vi "DI Scope.vi"(8 "error in (no error)":errorcluster, 11 "Node Ptr":T3 format="%.0x") -> (0 "error out":errorcluster)   [LabVIEW 2016, in "DCM System Explorer.lvlib"]
uses:
  DCM System Explorer.lvlib
  <vilib>/NI Veristand/Custom Device API/Custom Device Item Ref.ctl
  <vilib>/Powertrain Controls/Device Drivers/DCM/Rev0/FPGA/DI - ADC Signals.ctl
  <vilib>/Powertrain Controls/Device Drivers/DCM/DI/FPGA/Capture Event.ctl
  Shared/DCM Constants and GUIDs.vi
  <vilib>/NI Veristand/Custom Device Tools/Custom Device Utility Library/NI VeriStand - Search for Item by Name.vi
  <vilib>/NI VeriStand/Custom Device API/Custom Device API.lvlib
  DCM Shared.lvlib
  <vilib>/NI Veristand/Custom Device Tools/Custom Device Utility Library/Custom Device Utility Library.lvlib
  <vilib>/Powertrain Controls/Device Drivers/DCM/Rev0/FPGA/DCM - FPGA.lvlib
  <vilib>/Powertrain Controls/Device Drivers/DCM/DI/FPGA/DCM - FPGA - DI.lvlib
panel:
  in  "Capture Length":dbl caption="[s]"
  in  "Capture Enable":bool
  in  "Capture Event":T1
  in  "DI-ADC4-Select":T2 caption="Channel Select 4"
  in  "DI-ADC3-Select":T2 caption="Channel Select 3"
  in  "DI-ADC2-Select":T2 caption="Channel Select 2"
  in  "DI-ADC1-Select":T2 caption="Channel Select 1"
  in  "Header":cluster{"Section Name":string}={"Section Name"="DI Scope Initial Settings"}
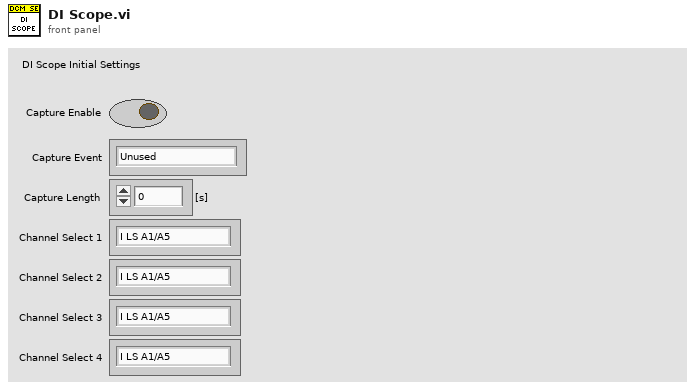
[diagram p1: front panel]
types:
  T1 = typedef "DCM - FPGA - DI.lvlib/Capture Event.ctl" = enum8{"Unused", "Injector A1", "Injector A2", "Injector A3", "Injector A4", "Injector A5", "Injector A6", "Injector A7", "Injector A8/PumpA", "Injector B1", "Injector B2", "Injector B3", "Injector B4", "Injector B5", "Injector B6", "Injector B7", "Injector B8/PumpB", "User OS", "Diff IO 1", "Diff IO 2", "Diff IO 3", "Diff IO 4", "Diff IO 5", "Diff IO 6", "Diff IO 7", "Diff IO 8", "Aux 1", "Aux 2", "Aux 3", "Aux 4", "Aux 5", "Aux 6", "Aux 7", "Aux 8", "Aux 9", "Aux 10", "Aux 11", "Aux 12", "Aux 13", "Aux 14", "Aux 15", "Aux 16"}
  T2 = typedef "DCM - FPGA.lvlib/DI - ADC Signals.ctl" = enum8{"I LS A1/A5", "I LS A2/A6", "I LS A3/A7", "I LS A4", "I LS A8/PumpA", "V PZ A1", "V PZ A2", "V PZ A3", "V PZ A4", "V S A1", "V S A2", "V S A3", "V S A4", "V S A5", "V S A6", "V S A7", "V S A8", "V Pump A", "V Secondary A1A2", "V Secondary A3A4", "V Ext HV A", "------------------------ ", "I LS B1/B5", "I LS B2/B6", "I LS B3/B7", "I LS B4", "I LS B8/PumpB", "V PZ B1", "V PZ B2", "V PZ B3", "V PZ B4", "V S B1", "V S B2", "V S B3", "V S B4", "V S B5", "V S B6", "V S B7", "V S B8", "V Pump B", "V Secondary B1B2", "V Secondary B3B4", "V Ext HV B", "-------------------------  ", "AI 1", "AI 2", "AI 3", "AI 4", "AI 5", "AI 6", "AI 7", "AI 8", "AI 9", "AI 10", "AI 11", "AI 12", "-------------------------   ", "V DRVP"}
  T3 = typedef "Custom Device API.lvlib/Custom Device Item Ref.ctl" = u64
  T4 = typedef "DCM Shared.lvlib/Channel.ctl" = cluster{"Name":string, "Units":string, "Default":dbl, "Description":string}
  T5 = typedef "Custom Device API.lvlib/Custom Device Channel.ctl" = cluster{"Type":T6, "Units":string, "Default Value":dbl, "Faultable":bool, "Scalable":bool}
  T6 = typedef "Custom Device API.lvlib/Custom Device Channel Type.ctl" = enum16{"Input", "Output"}
  T7 = typedef "Custom Device API.lvlib/Custom Device Commands.ctl" = enum16{"Default", "Item renamed", "Shutdown", "Dynamic button pressed"}
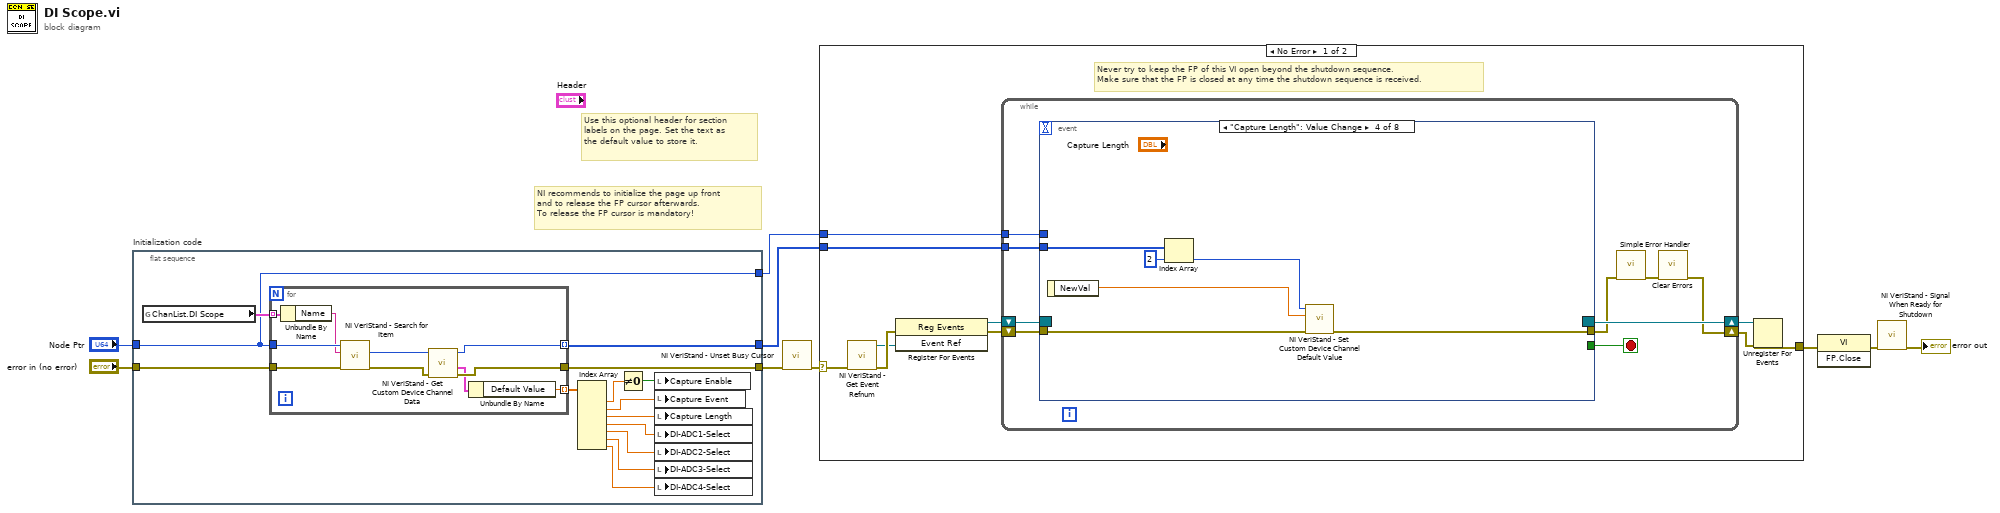
[diagram p0: block diagram]
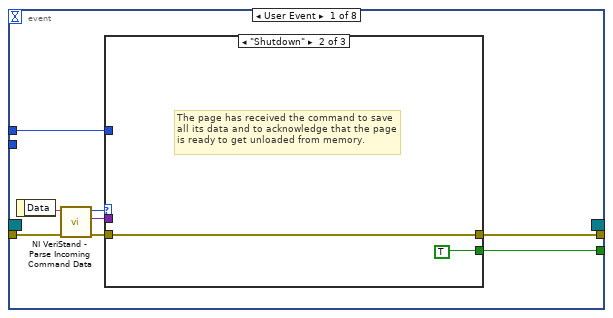
[diagram p2: hidden frame]
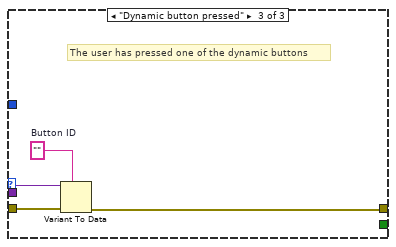
[diagram p4: hidden frame]
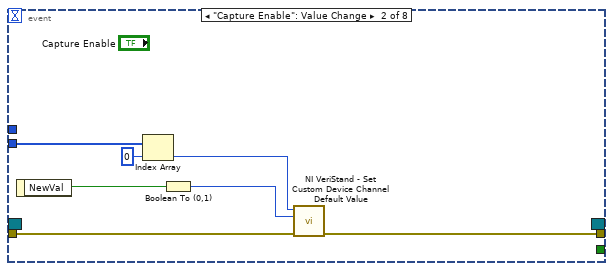
[diagram p5: hidden frame]
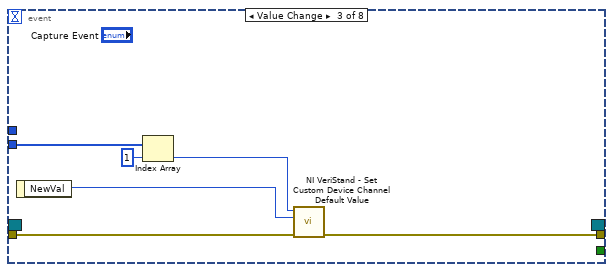
[diagram p6: hidden frame]
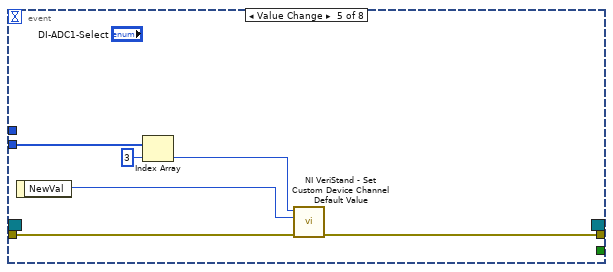
[diagram p7: hidden frame]
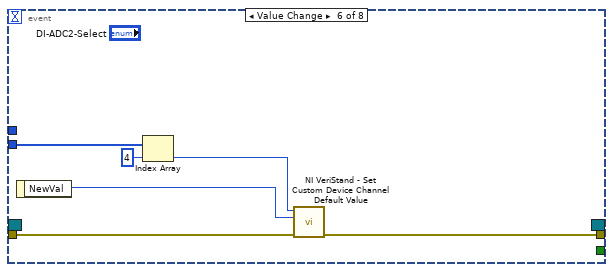
[diagram p8: hidden frame]
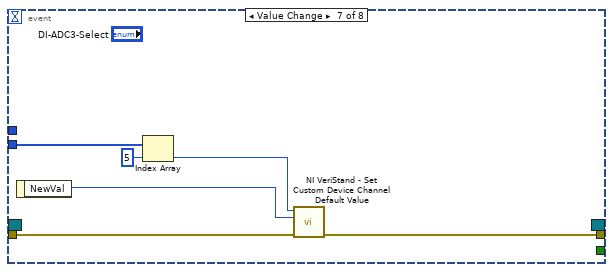
[diagram p9: hidden frame]
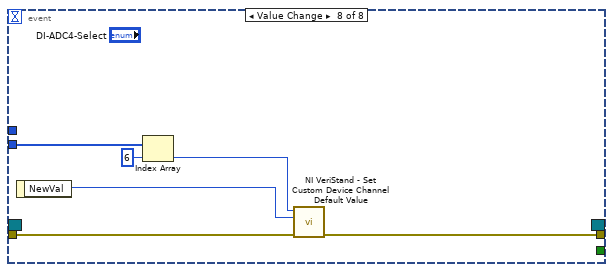
[diagram p10: hidden frame]
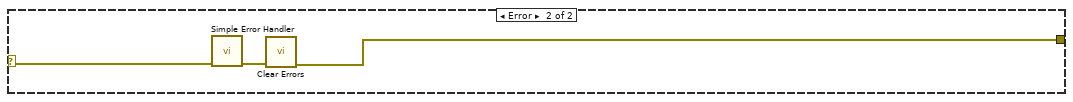
[diagram p11: hidden frame]
diagram:
  # "Use this optional header for section labels on the page. Set the text as the default value to store it."
  # "NI recommends to initialize the page up front\nand to release the FP cursor afterwards.\nTo release the FP cursor is mandatory!"
  n1 = flat-sequence "Initialization code" {
    tunnel: "error in (no error)" -> [w18]
    tunnel: "Node Ptr" -> [w16]
    tunnel: [w23] -> w5
    tunnel: [w17] -> w2
    tunnel: [w16] -> w1
    frame #0 {
      n2 = global read "DCM Constants and GUIDs.vi" "ChanList.DI Scope"() -> (w21:T4[])
      n3 = for {
        tunnel: w16 -> [w33]
        tunnel: w18 -> [w32]
        tunnel: [w24] -> w17 mode=indexing
        tunnel: [w30] -> w23
        tunnel: [w28] -> w22 mode=indexing
        tunnel: w21 -> [w27] mode=indexing
        n4 = Unbundle By Name(w27) -> ("Name"=w26:string)
        n5 = call-poly <vilib>:"NI VeriStand - Search for Item.vi"("error in"=w32, "Item Name"=w26, "Section Ref in"=w33) -> ("error out"=w31:errorcluster, "Item Ref"=w25:T3)  [unwired: 5 in, 2 out]
        n6 = call <vilib>:"NI VeriStand - Get Custom Device Channel Data.vi"("error in (no error)"=w31, "Channel Ref in"=w25) -> ("error out"=w30:errorcluster, "Channel"=w29:T5, "Channel Ref out"=w24:T3)  [unwired: 4 in, 3 out]
        n7 = Unbundle By Name(w29) -> ("Default Value"=w28:dbl)
      }
      n8 = Index Array(array=w22) -> (element #1=w12:dbl, element #2=w11:dbl, element #3=w10:dbl, element #4=w13:dbl, element #5=w15:dbl, element #6=w20:dbl, element #7=w19:dbl)  [unwired: 7 in]
      n9 = Not Equal To 0?(x=w12) -> (x != 0?=w14:bool)
      n10 = local write "Capture Enable"(w14) -> ()
      n11 = local write "Capture Event"(w11) -> ()
      n12 = local write "Capture Length"(w10) -> ()
      n13 = local write "DI-ADC1-Select"(w13) -> ()
      n14 = local write "DI-ADC2-Select"(w15) -> ()
      n15 = local write "DI-ADC3-Select"(w20) -> ()
      n16 = local write "DI-ADC4-Select"(w19) -> ()
    }
  }
  n17 = call <vilib>:"NI VeriStand - Unset Busy Cursor.vi"("error in (no error)"=w5) -> ("error out"=w4:errorcluster)  [unwired: 10 out]
  n18 = case shown="No Error" w4 {
    selector: w4 -> [w35 w113]
    tunnel: [w40 w111] -> w9
    tunnel: w2 -> [w36 _]
    tunnel: w1 -> [w34 _]
    frame No Error {
      # "Never try to keep the FP of this VI open beyond the shutdown sequence.\nMake sure that the FP is closed at any time the shutdown sequence is received."
      n19 = call <vilib>:"NI VeriStand - Get Event Refnum.vi"("error in (no error)"=w35) -> ("error out"=w43:errorcluster, "Event Ref"=w39:refnum<user-event>)  [unwired: 9 out]
      n20 = register-events(error in=w43, w39) -> (reference out=w37:refnum<event-registration>, error out=w38:errorcluster)  [unwired: 1 in]
      n21 = while {
        tunnel: w36 -> [w48]
        shift-right: [w45] -> w41
        shift-left: w38 -> [w51]
        shift-right: [w52] -> w42
        shift-left: w37 -> [w50]
        tunnel: w34 -> [w44]
        stop <- w49 stop-if-true
        n22 = event shown="[3] \"Capture Length\": Value Change" {
          selector: w50 -> [_ _ _ _ _ _ _ _]
          dyn-events: [_ _ _ _ _ _ _ _] -> w52
          timeout: _ -> [_ _ _ _ _ _ _ _]
          tunnel: w51 -> [w60 w72 w78 w84 w90 w96 w102 w108]
          tunnel: [w56 _ _ _ _ _ _ _] -> w49
          tunnel: [w55 w74 w80 w86 w92 w98 w104 w110] -> w47
          tunnel: w48 -> [_ w71 w77 w83 w89 w95 w101 w107]
          tunnel: w44 -> [w53 _ _ _ _ _ _ _]
          event User Event {
            n23 = event-data() -> ("Data"=w59:string)  [unwired: 1 out]
            n24 = call <vilib>:"NI VeriStand - Parse Incoming Command Data.vi"("error in (no error)"=w60, "Incoming data"=w59) -> ("error out"=w58:errorcluster, "Outgoing data"=w54:variant, "Action"=w57:T7)  [unwired: 7 out]
            n25 = case shown="\"Shutdown\"" w57 {
              tunnel: w58 -> [w61 w62 w67]
              tunnel: [_ TRUE _] -> w56
              tunnel: [w61 w62 w64] -> w55
              tunnel: w54 -> [_ _ w66]
              tunnel: w53 -> [_ _ _]
              frame "Default", Default {
              }
              frame "Shutdown" {
                # "The page has received the command to save all its data and to acknowledge that the page is ready to get unloaded from memory."
              }
              frame "Dynamic button pressed" {
                w65 = ""  # Button ID
                # "The user has pressed one of the dynamic buttons"
                n26 = Variant To Data(error in=w67, type=w65, Variant=w66) -> (error out=w64:errorcluster)  [unwired: 1 out]
              }
            }
          }
          event "Capture Enable": Value Change {
            n27 = event-data() -> ("NewVal"=w73:bool)  [unwired: 1 out]
            n28 = Index Array(array=w71, index=0) -> (element=w69:T3)
            n29 = Boolean To (0,1)(Boolean=w73) -> (0, 1=w68:i16)
            n30 = call <vilib>:"NI VeriStand - Set Custom Device Channel Default Value.vi"("error in (no error)"=w72, "Default Value"=w68, "Channel Ref in"=w69) -> ("error out"=w74:errorcluster)  [unwired: 7 in, 1 out]
          }
          event Value Change {
            n31 = event-data() -> ("NewVal"=w79:T1)  [unwired: 1 out]
            n32 = Index Array(array=w77, index=1) -> (element=w75:T3)
            n33 = call <vilib>:"NI VeriStand - Set Custom Device Channel Default Value.vi"("error in (no error)"=w78, "Default Value"=w79, "Channel Ref in"=w75) -> ("error out"=w80:errorcluster)  [unwired: 7 in, 1 out]
          }
          event "Capture Length": Value Change {
            n34 = event-data() -> ("NewVal"=w85:dbl)  [unwired: 1 out]
            n35 = Index Array(array=w83, index=2) -> (element=w81:T3)
            n36 = call <vilib>:"NI VeriStand - Set Custom Device Channel Default Value.vi"("error in (no error)"=w84, "Default Value"=w85, "Channel Ref in"=w81) -> ("error out"=w86:errorcluster)  [unwired: 7 in, 1 out]
          }
          event Value Change {
            n37 = event-data() -> ("NewVal"=w91:T2)  [unwired: 1 out]
            n38 = Index Array(array=w89, index=3) -> (element=w87:T3)
            n39 = call <vilib>:"NI VeriStand - Set Custom Device Channel Default Value.vi"("error in (no error)"=w90, "Default Value"=w91, "Channel Ref in"=w87) -> ("error out"=w92:errorcluster)  [unwired: 7 in, 1 out]
          }
          event Value Change {
            n40 = event-data() -> ("NewVal"=w97:T2)  [unwired: 1 out]
            n41 = Index Array(array=w95, index=4) -> (element=w93:T3)
            n42 = call <vilib>:"NI VeriStand - Set Custom Device Channel Default Value.vi"("error in (no error)"=w96, "Default Value"=w97, "Channel Ref in"=w93) -> ("error out"=w98:errorcluster)  [unwired: 7 in, 1 out]
          }
          event Value Change {
            n43 = event-data() -> ("NewVal"=w103:T2)  [unwired: 1 out]
            n44 = Index Array(array=w101, index=5) -> (element=w99:T3)
            n45 = call <vilib>:"NI VeriStand - Set Custom Device Channel Default Value.vi"("error in (no error)"=w102, "Default Value"=w103, "Channel Ref in"=w99) -> ("error out"=w104:errorcluster)  [unwired: 7 in, 1 out]
          }
          event Value Change {
            n46 = event-data() -> ("NewVal"=w109:T2)  [unwired: 1 out]
            n47 = Index Array(array=w107, index=6) -> (element=w105:T3)
            n48 = call <vilib>:"NI VeriStand - Set Custom Device Channel Default Value.vi"("error in (no error)"=w108, "Default Value"=w109, "Channel Ref in"=w105) -> ("error out"=w110:errorcluster)  [unwired: 7 in, 1 out]
          }
        }
        n49 = call <vilib>:"Simple Error Handler.vi"("error in (no error)"=w47) -> ("error out"=w46:errorcluster)  [unwired: 1 in, 7 out]
        n50 = call <vilib>:"Clear Errors.vi"("error in (no error)"=w46) -> ("error out"=w45:errorcluster)  [unwired: 1 in, 5 out]
      }
      n51 = Unregister For Events(event registration refnum=w42, error in=w41) -> (error out=w40:errorcluster)
    }
    frame Error {
      n52 = call <vilib>:"Simple Error Handler.vi"("error in (no error)"=w113) -> ("error out"=w112:errorcluster)  [unwired: 1 in, 7 out]
      n53 = call <vilib>:"Clear Errors.vi"("error in (no error)"=w112) -> ("error out"=w111:errorcluster)  [unwired: 1 in, 5 out]
    }
  }
  n54 = invoke class="VI" method="FP.Close"(error in=w9) -> (error out=w8:errorcluster)  [unwired: 2 in, 2 out]
  n55 = call <vilib>:"NI VeriStand - Signal When Ready for Shutdown.vi"("error in (no error)"=w8) -> ("error out"=→"error out":errorcluster)  [unwired: 10 out]
